vi "Fail.vi"(7 "Description":string, 8 "error in (no error)":errorcluster, 9 "Message":string, 11 "LUnit Test Case In":refnum<class "LUnit Test Case.lvclass">) -> (0 "error out":errorcluster, 3 "LUnit Test Case Out":refnum<class "LUnit Test Case.lvclass">)   [LabVIEW 2020, in "LUnit Test Case.lvclass"]
doc: "Generates a fail result for the calling test method. A description and message may be provided."
uses:
  LUnit Test Case.lvclass
  Result Classes/Assertion Result/Public/TypeDefs/Assertion Type.ctl
  LUnit Test Case.lvclass/LUnit Test Case.ctl
  Result Classes/Assertion Result/Assertion Result.lvclass/Assertion Result.ctl
  Result Classes/Test Case Result/Test Case Result.lvclass/Test Case Result.ctl
  Result Classes/Method Result/Method Result.lvclass/Method Result.ctl
  Result Classes/Test Case Result/Community/Record Assertion Result.vi
  Result Classes/Assertion Result/Community/Write Assertion Type.vi
  Result Classes/Method Result/Community/Accessors/Aggregate Assertion Results.vi
  Result Classes/Assertion Result/Public/Read Status.vi
  Result Classes/Assertion Result/Public/Read Message.vi
  Result Classes/Assertion Result/Public/Read Description.vi
  Result Classes/Method Result/Private/SubVIs/Merge Status.vi
  Result Classes/Method Result/Private/SubVIs/Concatenate result strings.vi
  Result Classes/Assertion Result/Assertion Result.lvclass
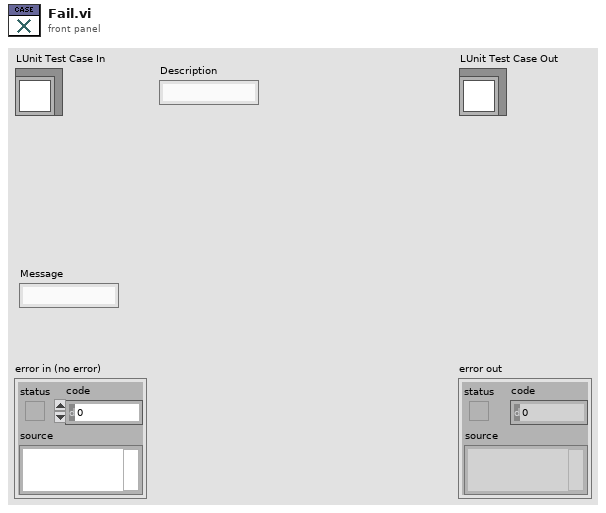
[diagram p1: front panel]
types:
  T1 = typedef "Assertion Result.lvclass/Assertion Type.ctl" = enum16{"None", "Pass", "Fail", "Skip", "Pass if Equal", "Fail if Equal", "Pass if Error", "Fail if Error", "Pass if", "Fail if"}
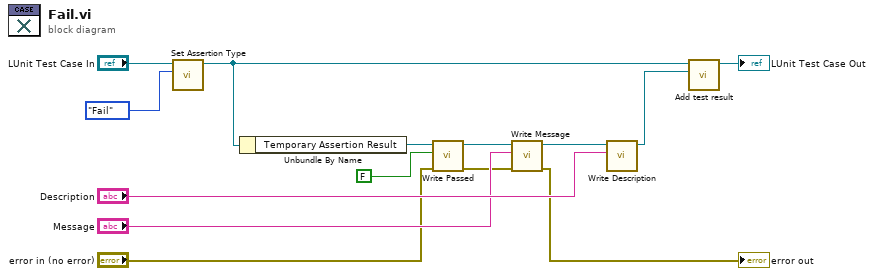
[diagram p0: block diagram]
diagram:
  n1 = call "Set Assertion Type.vi"("Assertion Type"=Assertion_Type."Fail", "LUnit Test Case In"="LUnit Test Case In") -> ("LUnit Test Case Out"=w7:refnum<class "LUnit Test Case.lvclass">)  [unwired: 9 in]
  n2 = Unbundle By Name(w7) -> ("Temporary Assertion Result"=w10:refnum<class "Assertion Result.lvclass">)
  n3 = call "Write Passed.vi"("error in (no error)"="error in (no error)", "Passed?"=FALSE, "Assertion Result In"=w10) -> ("error out"=w4:errorcluster, "Assertion Result Out"=w3:refnum<class "Assertion Result.lvclass">)  [unwired: 7 in]
  n4 = call "Write Message.vi"("error in (no error)"=w4, "Message"="Message", "Assertion Result In"=w3) -> ("error out"=→"error out":errorcluster, "Assertion Result Out"=w2:refnum<class "Assertion Result.lvclass">)  [unwired: 7 in]
  n5 = call "Write Description.vi"("Description"="Description", "Assertion Result In"=w2) -> ("Assertion Result Out"=w1:refnum<class "Assertion Result.lvclass">)  [unwired: 9 in]
  n6 = call "Add test result.vi"("Test Result"=w1, "LUnit Test Case In"=w7) -> ("LUnit Test Case Out"=→"LUnit Test Case Out":refnum<class "LUnit Test Case.lvclass">)  [unwired: 9 in]
